vi "Robot States.vi"() -> ()   [LabVIEW 2018]
panel:
  out "Elevator_State":string
  in  "Lower_Pulse_State":bool
  in  "Lower_Valve_State":bool
  in  "Upper_Pulse_State":bool
  in  "Upper_Valve_State":bool
  in  "HATCH_Ejection_Allowed":bool
  in  "HATCH_Ejection":bool
  in  "HATCH_Arm":bool
  in  "CARGO_Arm":bool
  in  "CARGO_Intake_Allowed":bool
  in  "Auto_Stow":bool
  in  "Autopilot":bool
  in  "Elevator_Brake_State":bool
  in  "Shifter_State":bool
  in  "Butterfly_State":bool
  # "Add Elevator State"
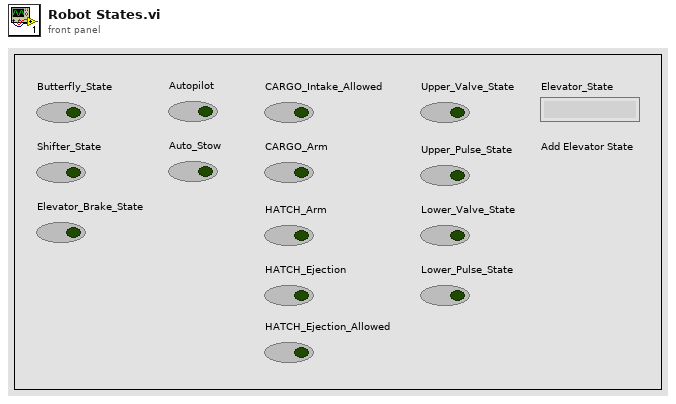
[diagram p1: front panel]
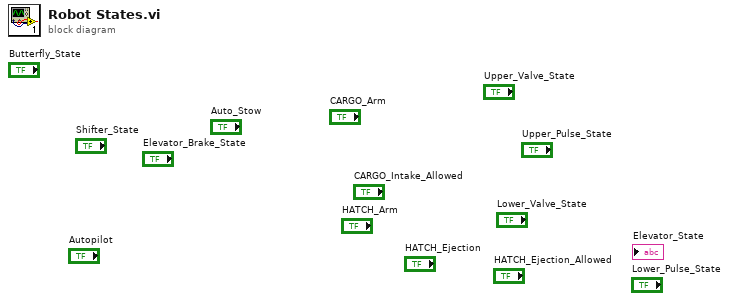
[diagram p0: block diagram]
diagram:
